vi "VI 1.vi"() -> ()   [LabVIEW 2020]
panel:
  in  "stop":bool
  out "x+y":dbl
  in  "y":dbl
  in  "x":dbl
  # "created VI"
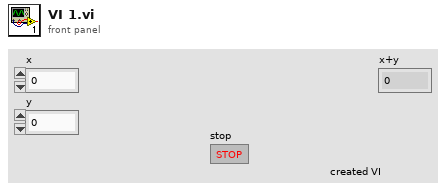
[diagram p1: front panel]
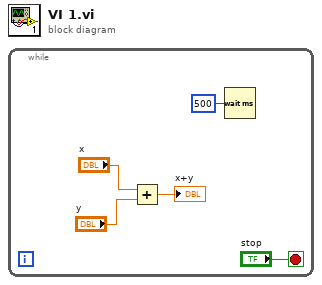
[diagram p0: block diagram]
diagram:
  n1 = while {
    stop <- "stop" stop-if-true
    n2 = Add(x="x", y="y") -> (x+y=→"x+y":dbl)
    n3 = Wait (ms)(milliseconds to wait=u32 500) -> ()  [unwired: 1 out]
  }
